vi "Average.vi"(0 "VISA IN":refnum<visa-resource-name>, 2 "AVG":i32, 5 "error in":errorcluster, 7 "Channel":i32=1) -> (14 "VISA Out":refnum<visa-resource-name>, 19 "error out":errorcluster)   [LabVIEW 2018, in "PNA-X.lvlib"]
uses:
  PNA-X.lvlib
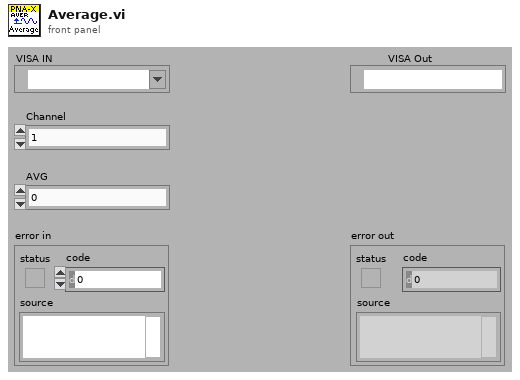
[diagram p1: front panel]
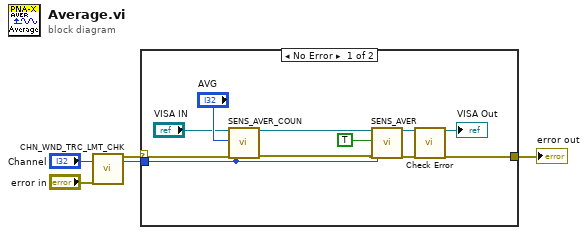
[diagram p0: block diagram]
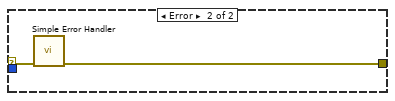
[diagram p2: hidden frame]
diagram:
  n1 = call "CHN_WND_TRC_LMT_CHK.vi"("Channel"="Channel", "error in"="error in") -> ("error out"=w2:errorcluster, "Channel"=w1:i32)  [unwired: 13 in, 3 out]
  n2 = case shown="No Error" w2 {
    selector: w2 -> [w12 w18]
    tunnel: [w15 w17] -> w4
    tunnel: w1 -> [w7 _]
    frame No Error {
      n3 = call "SENS_AVER_COUN.vi"("VISA IN"="VISA IN", "AVG"="AVG", "error in"=w12, "Channel"=w7) -> ("VISA Out"=w10:refnum<visa-resource-name>, "error out"=w6:errorcluster)  [unwired: 14 in]
      n4 = call "SENS_AVER.vi"("VISA IN"=w10, "Average ON/OFF"=TRUE, "error in"=w6, "Channel"=w7) -> ("VISA Out"=w9:refnum<visa-resource-name>, "error out"=w11:errorcluster)  [unwired: 14 in]
      n5 = call "Check Error.vi"("VISA Resource Name"=w9, "error in (no error)"=w11) -> ("dup VISA session"=→"VISA Out":refnum<visa-resource-name>, "error out"=w15:errorcluster)  [unwired: 16 in]
    }
    frame Error {
      n6 = call <vilib>:"Simple Error Handler.vi"("error in (no error)"=w18) -> ("error out"=w17:errorcluster)  [unwired: 4 in, 4 out]
    }
  }
  "error out" <- w4
